vi "Insert into Service Map.vi"(8 "error in":errorcluster, 10 "COB-ID":u32 format="%.0x", 11 "CANopen in":refnum<class "CANopen.lvclass">) -> (0 "error out":errorcluster, 2 "Notifier":refnum<notifier>, 3 "CANopen out":refnum<class "CANopen.lvclass">)   [LabVIEW 2026, in "canopen_.lvlib" / "CANopen.lvclass"]
doc: "Appends a new entry inside the service map. The insertion is protected by a mutex in order to prevent race conditions with \"Service map delete\"."
uses:
  CANopen.lvclass
  CANopen.lvclass/CANopen.ctl
  <vilib>/Utility/miscctls.llb/LVMapReplaceAction.ctl
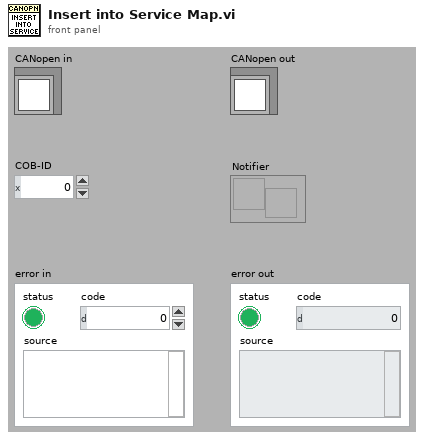
[diagram p1: front panel]
types:
  T1 = typedef "LVMapReplaceAction.ctl" = enum32{"Modify Entry only if found", "Add or Modify Entry", "Delete Entry"}
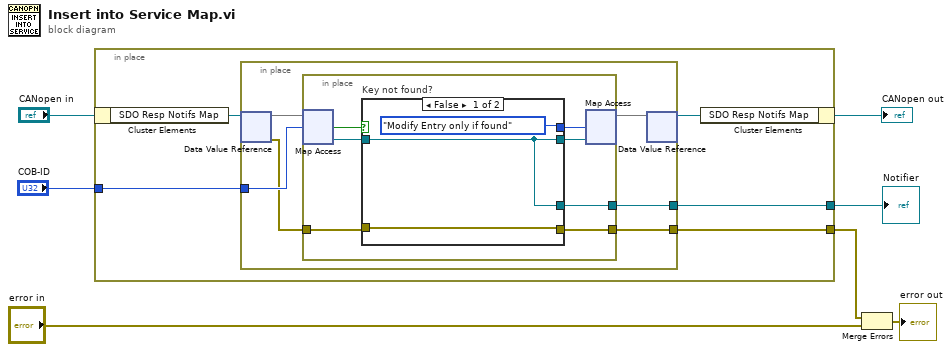
[diagram p0: block diagram]
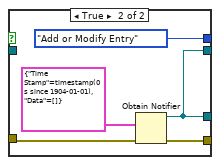
[diagram p2: hidden frame]
diagram:
  n1 = in-place {
    in-place-border: "COB-ID" -> [w12]
    in-place-border: [w9] -> w3
    in-place-border: [w8] -> w1
    n2 = in-place-cluster #1("CANopen in") -> ("SDO Resp Notifs Map"=w10:refnum<data-value>)
    n3 = in-place {
      in-place-border: w12 -> [w17]
      in-place-border: [w14] -> w9
      in-place-border: [w13] -> w8
      n4 = in-place-dvr #2(w10) -> (w18:map{u32, refnum<notifier>}, w16:errorcluster)
      n5 = in-place {
        in-place-border: w16 -> [w25]
        in-place-border: [w20] -> w14
        in-place-border: [w19] -> w13
        n6 = in-place-map #3(w18, w17) -> (w21:refnum<notifier>, w22:bool)  [unwired: 1 in]
        n7 = case "Key not found?" shown="False" w22 {
          tunnel: w25 -> [w27 w32]
          tunnel: [LVMapReplaceAction."Modify Entry only if found" ("action") LVMapReplaceAction."Add or Modify Entry" ("action")] -> w24
          tunnel: [w26 w29] -> w23
          tunnel: w21 -> [w26 _]
          tunnel: [w27 w30] -> w20
          tunnel: [w26 w29] -> w19
          frame False {
          }
          frame True {
            n8 = Obtain Notifier(notification data type=cluster{"Time Stamp":timestamp, "Data":u8[]} {"Time Stamp"=timestamp(0 s since 1904-01-01), "Data"=[]} ("CAN Msg received"), error in (no error)=w32) -> (notifier out=w29:refnum<notifier>, error out=w30:errorcluster)  [unwired: 2 in, 1 out]
          }
        }
        n9 = in-place-map #3(w23, w24) -> (w15:map{u32, refnum<notifier>})  [unwired: 2 out]
      }
      n10 = in-place-dvr #2(w15) -> (w11:refnum<data-value>)  [unwired: 1 out]
    }
    n11 = in-place-cluster #1("SDO Resp Notifs Map"=w11) -> (→"CANopen out":refnum<class "CANopen.lvclass">)
  }
  "Notifier" <- w1
  n12 = Merge Errors(w3, "error in") -> (→"error out":errorcluster)
